vi "Copy Linked List.vi"(5 "Recursive? (T)":bool=TRUE, 6 "Insertion Index":i32=-1, 7 "New Parent Linked List ID":string, 8 "error in (no error)":errorcluster, 9 "New Linked List ID":string, 10 "Linked List ID":string, 11 "Linked List in":refnum<class "Linked List.lvclass">) -> (0 "error out":errorcluster, 2 "Linked List ID out":string, 3 "Linked List out":refnum<class "Linked List.lvclass">, 4 "Children":string[](array[string]))   [LabVIEW 2020, in "Linked Lists.lvlib" / "Linked List.lvclass"]
uses:
  <vilib>/gpm_packages/@cs/linked-list/Source/Linked List/Linked List/Linked List.lvclass
  <vilib>/gpm_packages/@cs/linked-list/Source/Linked List/Linked List Definition/Linked List Definition.lvclass
  <vilib>/gpm_packages/@cs/linked-list/Source/Linked List/Linked List/Linked List.lvclass/Linked List.ctl
  <vilib>/gpm_packages/@cs/lookup-table/Source/LookupTable/LookupTable.lvclass/LookupTable.ctl
  dea0f38d-61f3-466e-aa12-9ceaa26f2994.vi
  <vilib>/gpm_packages/@cs/lookup-table/Source/LookupTable/Read Table Reference.vi
  dea0f38d-61f3-466e-aa12-9ceaa26f2994.vi/5a7267ad-595e-4610-9ac2-8bef780848ff.vi
  <vilib>/gpm_packages/@cs/lookup-table/Source/LookupTable/LookupTable.lvclass
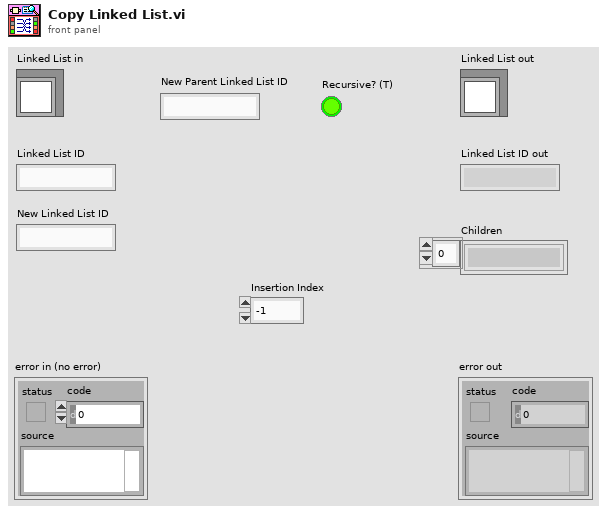
[diagram p1: front panel]
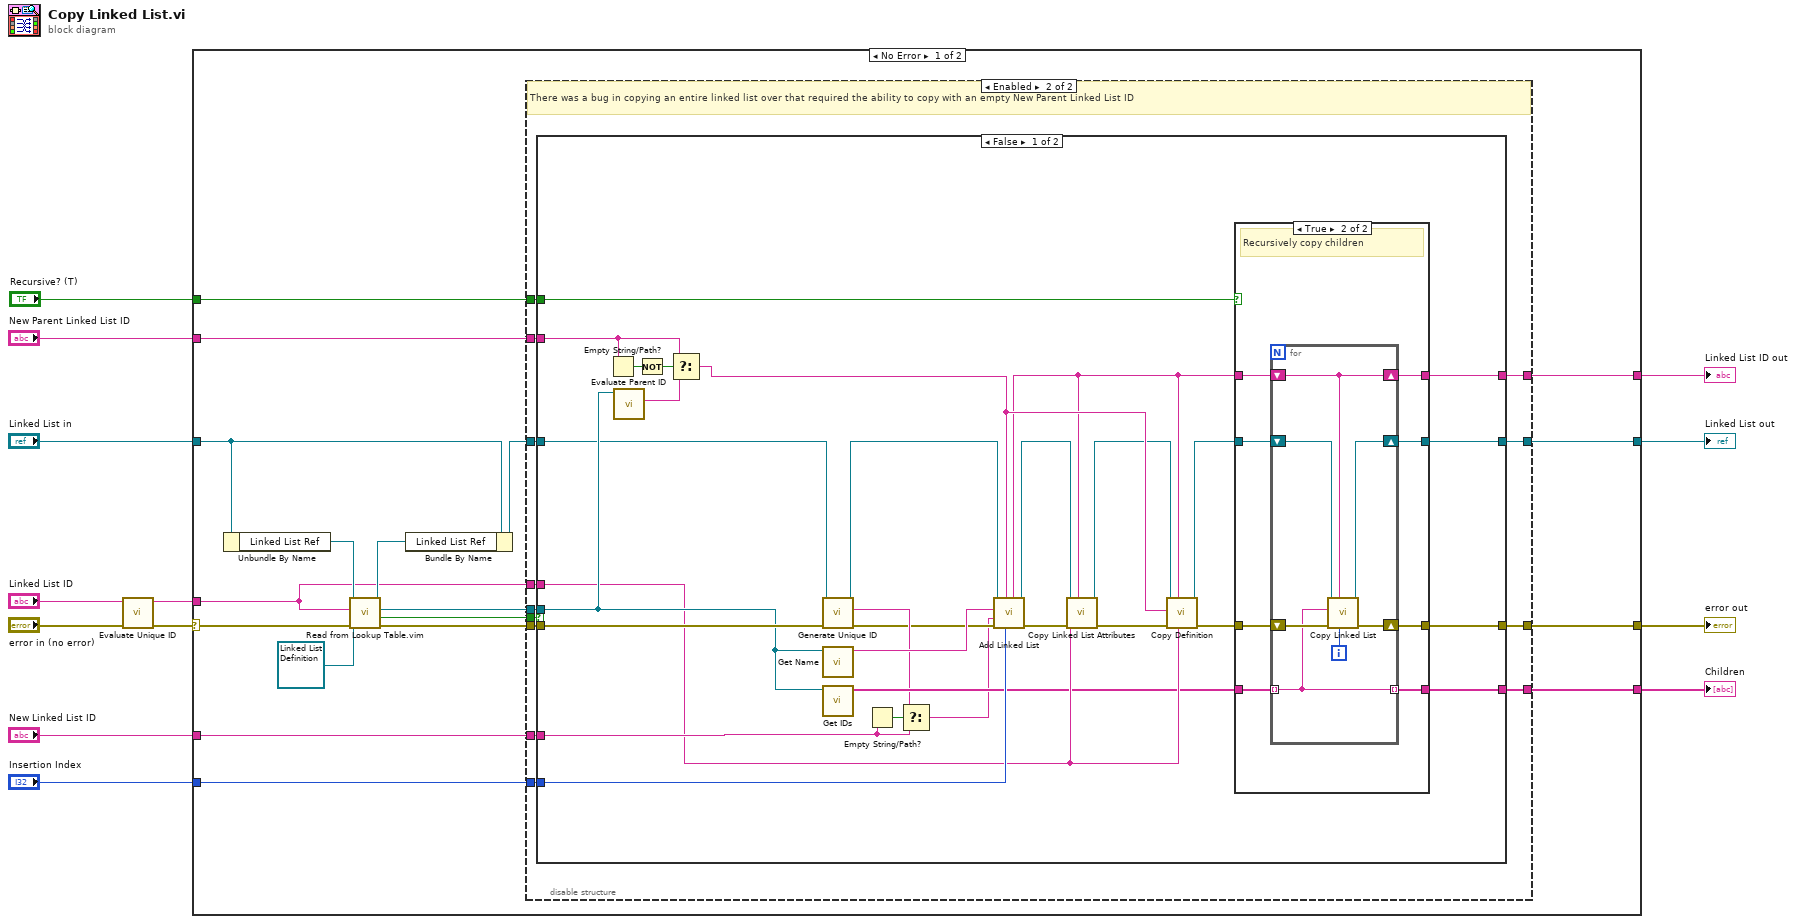
[diagram p0: block diagram]
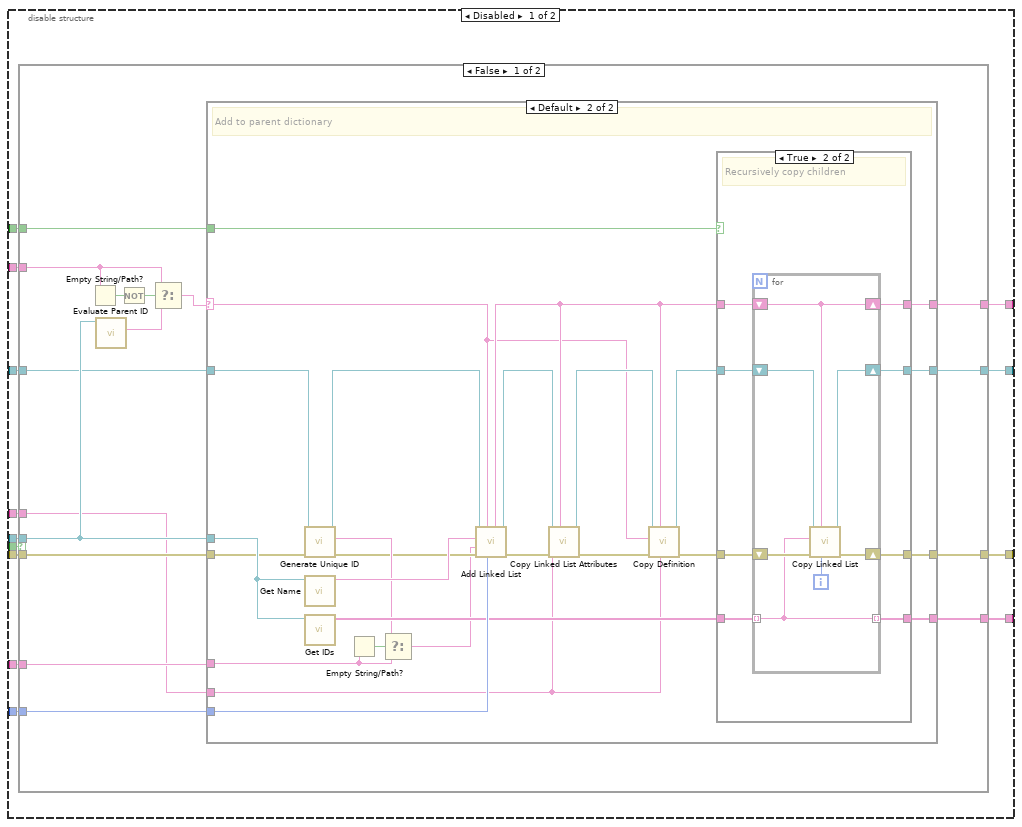
[diagram p2: hidden frame]
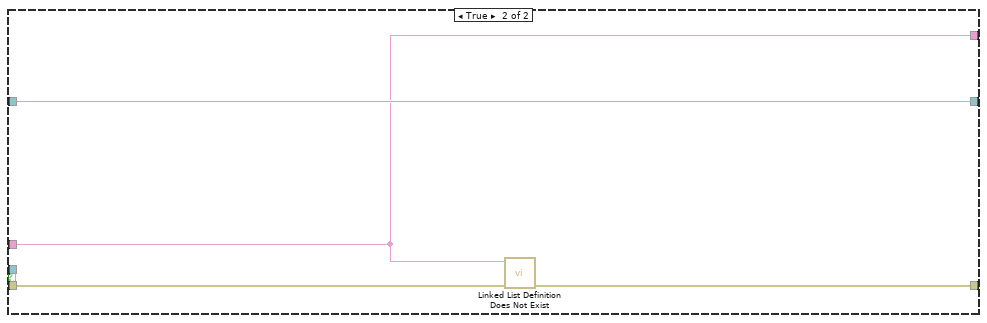
[diagram p5: hidden frame]
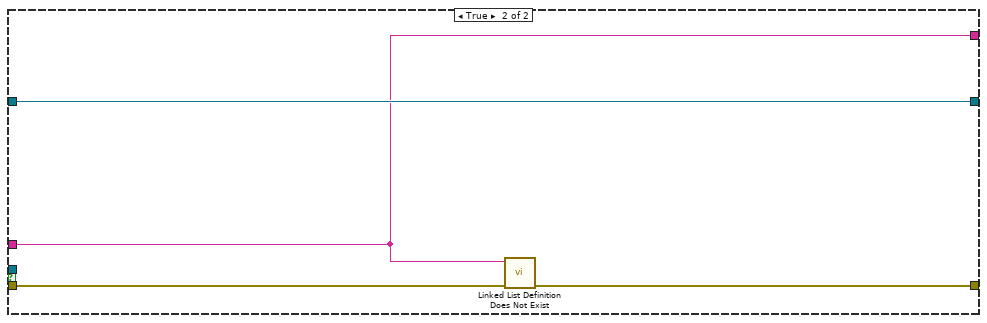
[diagram p7: hidden frame]
diagram:
  n1 = call <vilib>:"Evaluate Unique ID.vi"("error in (no error)"="error in (no error)", "Unique ID"="Linked List ID") -> ("error out"=w11:errorcluster, "Unique ID Out"=w10:string)  [unwired: 8 in]
  n2 = case shown="No Error" w11 {
    selector: w11 -> [w29 w179]
    tunnel: w10 -> [w17 _]
    tunnel: "Linked List in" -> [w25 w180]
    tunnel: "New Linked List ID" -> [w23 _]
    tunnel: [w22 w180] -> w7
    tunnel: [w21 w179] -> w6
    tunnel: "New Parent Linked List ID" -> [w20 _]
    tunnel: "Insertion Index" -> [w19 _]
    tunnel: [w18 _] -> w3
    tunnel: "Recursive? (T)" -> [w15 _]
    tunnel: [w14 _] -> w1
    frame No Error {
      n3 = Unbundle By Name(w25) -> ("Linked List Ref"=w31:refnum<data-value>)
      n4 = call "Read from Lookup Table.vim"("error in (no error)"=w29, "Type"=refnum<class "Linked List Definition.lvclass"> refnum ("Linked List.lvlib:Linked List Definition.lvclass"), "Item Name"=w17, "LookupTable Reference"=w31) -> ("error out"=w28:errorcluster, "Not Found?"=w16:bool, "Value"=w27:refnum<class "Linked List Definition.lvclass">, "LookupTable Reference Out"=w26:refnum<data-value>)  [unwired: 4 in]
      n5 = Bundle By Name(cluster=w25, "Linked List Ref"=w26) -> (w24:refnum<class "Linked List.lvclass">)
      n6 = disable-structure shown="Enabled" {
        disable-tunnel: w28 -> [w44 w125]
        disable-tunnel: w27 -> [w43 w124]
        disable-tunnel: w24 -> [w42 w123]
        disable-tunnel: w23 -> [w41 w122]
        disable-tunnel: [w40 w121] -> w22
        disable-tunnel: [w39 w120] -> w21
        disable-tunnel: w20 -> [w38 w119]
        disable-tunnel: w19 -> [w37 w118]
        disable-tunnel: [w36 w117] -> w18
        disable-tunnel: w17 -> [w35 w116]
        disable-tunnel: w16 -> [w34 w115]
        disable-tunnel: w15 -> [w33 w114]
        disable-tunnel: [w32 w113] -> w14
        frame Disabled {
          n7 = case shown="False" w34 {
            tunnel: w44 -> [w60 w111]
            tunnel: w43 -> [w59 _]
            tunnel: w42 -> [w58 w112]
            tunnel: w41 -> [w57 _]
            tunnel: [w56 w112] -> w40
            tunnel: [w55 w110] -> w39
            tunnel: w38 -> [w54 _]
            tunnel: w37 -> [w53 _]
            tunnel: [w52 w109] -> w36
            tunnel: w35 -> [w51 w109]
            tunnel: w33 -> [w46 _]
            tunnel: [w45 _] -> w32
            frame False {
              n8 = Empty String/Path?(string/path=w54) -> (empty?=w50:bool)
              n9 = call <vilib>:"Evaluate Parent ID.vi"("Linked List Definition in"=w59) -> ("Parent ID"=w48:string)  [unwired: 8 in, 2 out]
              n10 = Not(x=w50) -> (.not. x?=w49:bool)
              n11 = Select(t=w54, s=w49, f=w48) -> (s? t:f=w47:string)
              n12 = case shown="Default" w47 {
                selector: w47 -> [w61 w67]
                tunnel: w60 -> [w62 w80]
                tunnel: [w62 w75] -> w55
                tunnel: w58 -> [w63 w78]
                tunnel: [w63 w76] -> w56
                tunnel: w51 -> [_ w66]
                tunnel: w53 -> [_ w89]
                tunnel: [w61 w83] -> w52
                tunnel: w59 -> [_ w85]
                tunnel: w57 -> [_ w74]
                tunnel: w46 -> [_ w65]
                tunnel: [_ w64] -> w45
                frame "" {
                  # "No parent, should never execute"
                }
                frame Default {
                  # "Add to parent dictionary"
                  n13 = call <vilib>:"Generate Unique ID.vi"("error in (no error)"=w80, "Linked List in"=w78) -> ("error out"=w79:errorcluster, "ID"=w82:string, "Linked List out"=w77:refnum<class "Linked List.lvclass">)  [unwired: 7 in]
                  n14 = call <vilib>:"Get Name.vi"("Linked List Definition in"=w85) -> ("Name"=w88:string)  [unwired: 8 in, 2 out]
                  n15 = call <vilib>:"Get IDs.vi"("Linked List Definition in"=w85) -> ("Child IDs"=w84:string[])  [unwired: 8 in, 2 out]
                  n16 = Empty String/Path?(string/path=w74) -> (empty?=w81:bool)
                  n17 = Select(t=w82, s=w81, f=w74) -> (s? t:f=w73:string)
                  n18 = call-dynamic "Add Linked List.vi"("Insertion Index"=w89, "Parent ID"=w67, "error in (no error)"=w79, "Unique ID"=w73, "Name"=w88, "Linked List in"=w77) -> ("error out"=w86:errorcluster, "Linked List out"=w87:refnum<class "Linked List.lvclass">, "Unique ID out"=w70:string)  [unwired: 2 in, 1 out]
                  n19 = call-dynamic "Copy Linked List Attributes.vi"("Sink Linked List ID"=w70, "error in (no error)"=w86, "Source Linked List ID"=w66, "Linked List in"=w87) -> ("error out"=w72:errorcluster, "Linked List out"=w69:refnum<class "Linked List.lvclass">)  [unwired: 6 in]
                  n20 = call-dynamic "Copy Definition.vi"("Source Linked List ID"=w66, "Sink Linked List ID"=w70, "error in (no error)"=w72, "Sink Parent Linked List ID"=w67, "Linked List in"=w69) -> ("error out"=w71:errorcluster, "Linked List out"=w68:refnum<class "Linked List.lvclass">)  [unwired: 5 in]
                  n21 = case shown="True" w65 {
                    tunnel: w84 -> [w90 w101]
                    tunnel: [w93 w100] -> w83
                    tunnel: [w92 w99] -> w76
                    tunnel: [w91 w98] -> w75
                    tunnel: w71 -> [w91 w97]
                    tunnel: w70 -> [w93 w96]
                    tunnel: w68 -> [w92 w95]
                    tunnel: [w90 w94] -> w64
                    frame False {
                    }
                    frame True {
                      # "Recursively copy children"
                      n22 = for {
                        shift-right: [w105] -> w98
                        shift-left: w97 -> [w106]
                        shift-right: [w107] -> w99
                        shift-left: w95 -> [w108]
                        tunnel: w101 -> [w102] mode=indexing
                        shift-right: [w104] -> w100
                        shift-left: w96 -> [w104]
                        tunnel: [w102] -> w94 mode=indexing
                        i -> [w103]
                        n23 = call-dynamic "Copy Linked List.vi"("Insertion Index"=w103, "New Parent Linked List ID"=w104, "error in (no error)"=w106, "Linked List ID"=w102, "Linked List in"=w108) -> ("error out"=w105:errorcluster, "Linked List out"=w107:refnum<class "Linked List.lvclass">)  [unwired: 3 in, 2 out]
                      }
                    }
                  }
                }
              }
            }
            frame True {
              n24 = call <vilib>:"Linked List Definition Does Not Exist.vi"("Error In"=w111, "Unique ID"=w109) -> ("Error Out"=w110:errorcluster)  [unwired: 9 in]
            }
          }
        }
        frame Enabled {
          # "There was a bug in copying an entire linked list over that required the ability to copy with an empty New Parent Linked List ID"
          n25 = case shown="False" w115 {
            tunnel: w125 -> [w155 w177]
            tunnel: w124 -> [w154 _]
            tunnel: w123 -> [w153 w178]
            tunnel: w122 -> [w152 _]
            tunnel: [w151 w178] -> w121
            tunnel: [w150 w176] -> w120
            tunnel: w119 -> [w149 _]
            tunnel: w118 -> [w148 _]
            tunnel: [w147 w175] -> w117
            tunnel: w116 -> [w146 w175]
            tunnel: w114 -> [w141 _]
            tunnel: [w140 _] -> w113
            frame False {
              n26 = Empty String/Path?(string/path=w149) -> (empty?=w145:bool)
              n27 = call <vilib>:"Evaluate Parent ID.vi"("Linked List Definition in"=w154) -> ("Parent ID"=w143:string)  [unwired: 8 in, 2 out]
              n28 = Not(x=w145) -> (.not. x?=w144:bool)
              n29 = Select(t=w149, s=w144, f=w143) -> (s? t:f=w142:string)
              n30 = call <vilib>:"Generate Unique ID.vi"("error in (no error)"=w155, "Linked List in"=w153) -> ("error out"=w133:errorcluster, "ID"=w135:string, "Linked List out"=w132:refnum<class "Linked List.lvclass">)  [unwired: 7 in]
              n31 = call <vilib>:"Get Name.vi"("Linked List Definition in"=w154) -> ("Name"=w139:string)  [unwired: 8 in, 2 out]
              n32 = call <vilib>:"Get IDs.vi"("Linked List Definition in"=w154) -> ("Child IDs"=w136:string[])  [unwired: 8 in, 2 out]
              n33 = Empty String/Path?(string/path=w152) -> (empty?=w134:bool)
              n34 = Select(t=w135, s=w134, f=w152) -> (s? t:f=w131:string)
              n35 = call-dynamic "Add Linked List.vi"("Insertion Index"=w148, "Parent ID"=w142, "error in (no error)"=w133, "Unique ID"=w131, "Name"=w139, "Linked List in"=w132) -> ("error out"=w137:errorcluster, "Linked List out"=w138:refnum<class "Linked List.lvclass">, "Unique ID out"=w128:string)  [unwired: 2 in, 1 out]
              n36 = call-dynamic "Copy Linked List Attributes.vi"("Sink Linked List ID"=w128, "error in (no error)"=w137, "Source Linked List ID"=w146, "Linked List in"=w138) -> ("error out"=w130:errorcluster, "Linked List out"=w127:refnum<class "Linked List.lvclass">)  [unwired: 6 in]
              n37 = call-dynamic "Copy Definition.vi"("Source Linked List ID"=w146, "Sink Linked List ID"=w128, "error in (no error)"=w130, "Sink Parent Linked List ID"=w142, "Linked List in"=w127) -> ("error out"=w129:errorcluster, "Linked List out"=w126:refnum<class "Linked List.lvclass">)  [unwired: 5 in]
              n38 = case shown="True" w141 {
                tunnel: w136 -> [w156 w167]
                tunnel: [w159 w166] -> w147
                tunnel: [w158 w165] -> w151
                tunnel: [w157 w164] -> w150
                tunnel: w129 -> [w157 w163]
                tunnel: w128 -> [w159 w162]
                tunnel: w126 -> [w158 w161]
                tunnel: [w156 w160] -> w140
                frame False {
                }
                frame True {
                  # "Recursively copy children"
                  n39 = for {
                    shift-right: [w171] -> w164
                    shift-left: w163 -> [w172]
                    shift-right: [w173] -> w165
                    shift-left: w161 -> [w174]
                    tunnel: w167 -> [w168] mode=indexing
                    shift-right: [w170] -> w166
                    shift-left: w162 -> [w170]
                    tunnel: [w168] -> w160 mode=indexing
                    i -> [w169]
                    n40 = call-dynamic "Copy Linked List.vi"("Insertion Index"=w169, "New Parent Linked List ID"=w170, "error in (no error)"=w172, "Linked List ID"=w168, "Linked List in"=w174) -> ("error out"=w171:errorcluster, "Linked List out"=w173:refnum<class "Linked List.lvclass">)  [unwired: 3 in, 2 out]
                  }
                }
              }
            }
            frame True {
              n41 = call <vilib>:"Linked List Definition Does Not Exist.vi"("Error In"=w177, "Unique ID"=w175) -> ("Error Out"=w176:errorcluster)  [unwired: 9 in]
            }
          }
        }
      }
    }
    frame Error {
    }
  }
  "error out" <- w6
  "Linked List out" <- w7
  "Linked List ID out" <- w3
  "Children" <- w1
